vi "Start Macro Recording.vi"(8 "error in (no error)":errorcluster, 10 "Start Macro (\"File\")":string="File", 11 "VISA resource name":refnum<visa-resource-name>) -> (0 "error out":errorcluster, 3 "VISA resource name out":refnum<visa-resource-name>)   [LabVIEW 2020, in "Rohde&Schwarz CMXP Base.lvlib"]
doc: "Starts recording of submitted commands into a macro file. If the file exists, it is overwritten. If the file does not exist, it is created.\n\nAttribute:\nRSCMXPBASE_ATTR_START_MACRO_RECORDING\n\nRemote-control command:\nSYSTem:RECord:MACRo:FILE:STARt"
uses:
  <instrlib>/Rohde&Schwarz CMXP Base/Rohde&Schwarz CMXP Base.lvlib
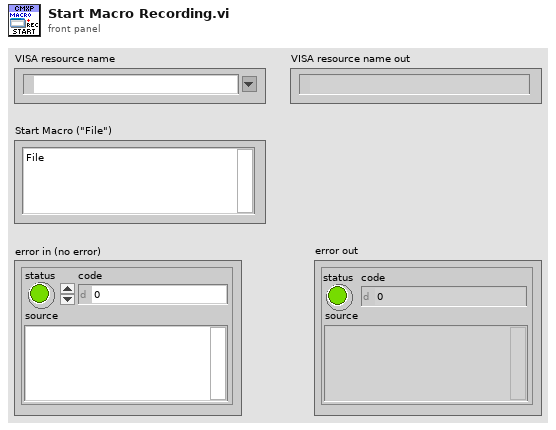
[diagram p1: front panel]
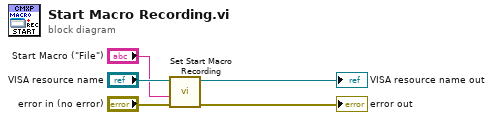
[diagram p0: block diagram]
diagram:
  n1 = call "Set Start Macro Recording"("error in (no error)"="error in (no error)", "Start Macro Recording ()"="Start Macro (\"File\")", "instrument handle"="VISA resource name") -> ("error out"=→"error out":errorcluster, "instrument handle out"=→"VISA resource name out":refnum<visa-resource-name>)  [unwired: 7 in]
